vi "LogStatus.vi"(7 "Station":enum16{"A", "B"}(ring), 8 "error in (no error)":errorcluster, 9 "last message":string, 10 "message":string) -> (0 "error  out":errorcluster)   [LabVIEW 2017]
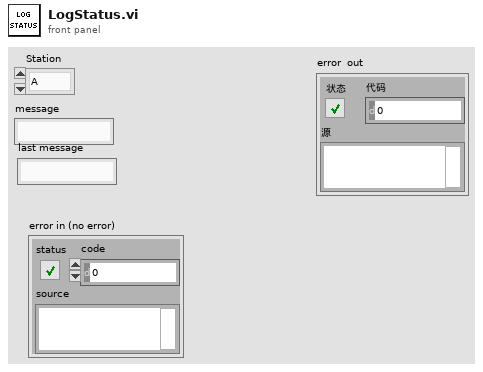
[diagram p1: front panel]
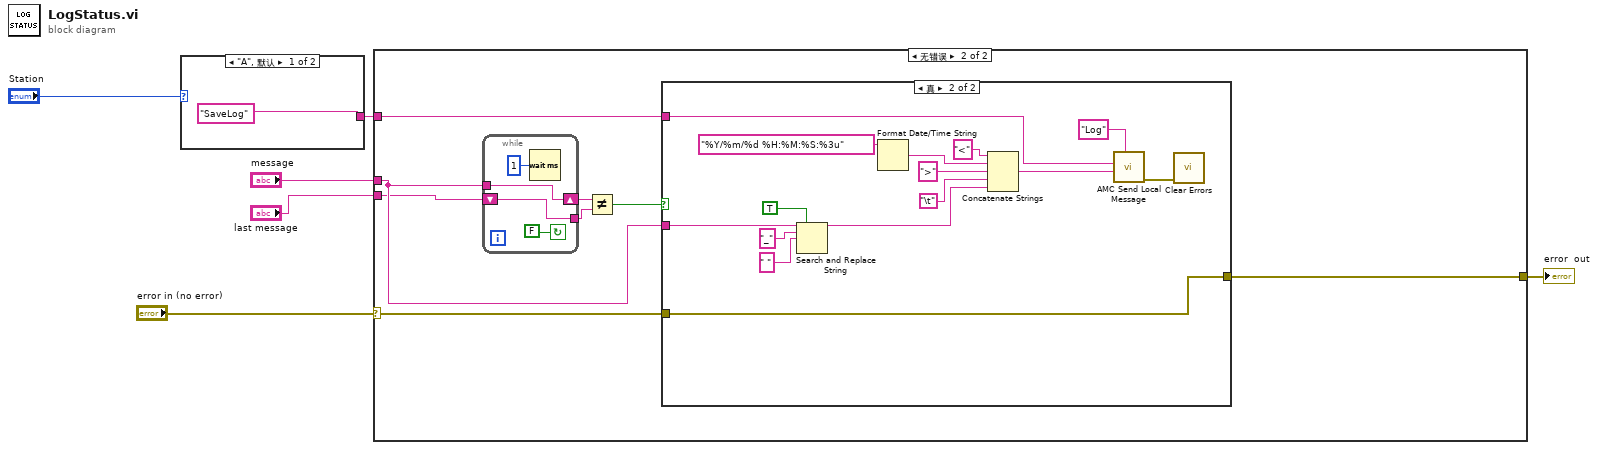
[diagram p0: block diagram]
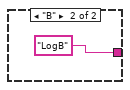
[diagram p2: hidden frame]
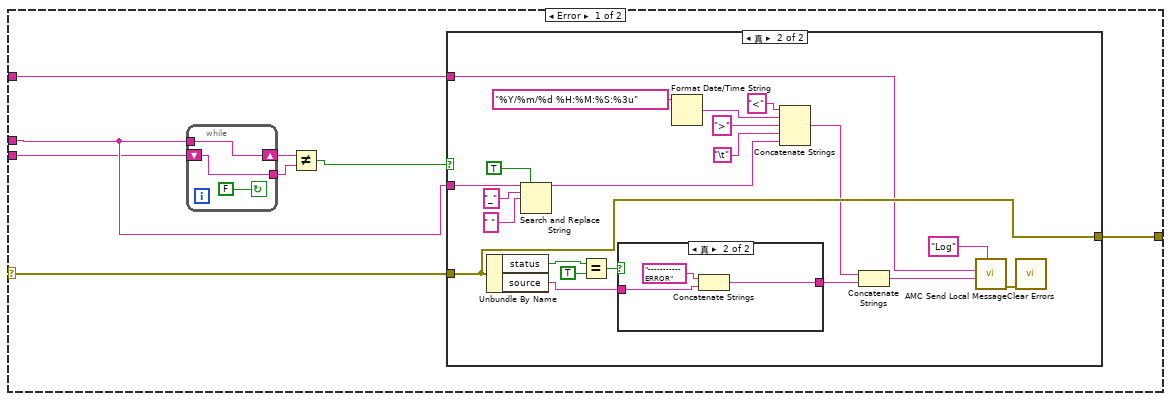
[diagram p3: hidden frame]
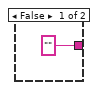
[diagram p5: hidden frame]
diagram:
  n1 = case shown="\"A\", 默认" "Station" {
    tunnel: ["SaveLog" ("Message Name") "LogB" ("Process (\"\" - local)")] -> w4
    frame "A", Default {
    }
    frame "B" {
    }
  }
  n2 = case shown="无错误" "error in (no error)" {
    selector: "error in (no error)" -> [w16 w53]
    tunnel: "message" -> [w11 w48]
    tunnel: [w15 w52] -> w6
    tunnel: w4 -> [w12 w51]
    tunnel: "last message" -> [w10 w47]
    frame Error {
      n3 = while {
        shift-right: [w19] -> w13
        shift-left: w10 -> [w18]
        tunnel: w11 -> [w19]
        tunnel: [w18] -> w14
        stop <- FALSE continue-if-true
      }
      n4 = Not Equal?(x=w13, y=w14) -> (x != y?=w9:bool)
      n5 = case shown="真" w9 {
        tunnel: w11 -> [_ w33]
        tunnel: w16 -> [w20 w32]
        tunnel: [w20 w32] -> w15
        tunnel: w12 -> [_ w22]
        frame False {
        }
        frame True {
          n6 = Unbundle By Name(w32) -> ("status"=w38:bool, "source"=w41:string)
          n7 = Search and Replace String(replace all?=TRUE ("替换全部？(F)"), input string=w33, search string="_" ("搜索字符串"), replace string=" " ("替换字符串(\"\")")) -> (result string=w25:string)  [unwired: 4 in, 3 out]
          n8 = Equal?(x=w38, y=TRUE) -> (x = y?=w40:bool)
          n9 = case shown="真" w40 {
            tunnel: ["" ("string") w44] -> w39
            tunnel: w41 -> [_ w43]
            frame False {
            }
            frame True {
              n10 = Concatenate Strings("-----------ERROR" ("string"), w43) -> (w44:string)
            }
          }
          n11 = Format Date/Time String(time format string (%c)="%Y/%m/%d %H:%M:%S:%3u" ("时间格式字符串(%c)")) -> (date/time string=w30:string)  [unwired: 2 in]
          n12 = Concatenate Strings("<" ("字符串"), w30, ">" ("字符串"), "\t", w25) -> (w24:string)
          n13 = Concatenate Strings(w24, w39) -> (w31:string)
          n14 = call "AMC Send Local Message.vi"("Process (\"\" - local)"="Log" ("Process (\"\" - local)"), "Message Value"=w31, "Message Name"=w22) -> ("error out"=w21:errorcluster)  [unwired: 7 in, 1 out]
          n15 = call <vilib>:"Clear Errors.vi"("error in (no error)"=w21) -> ()  [unwired: 5 in, 2 out]
        }
      }
    }
    frame No Error {
      n16 = while {
        shift-right: [w57] -> w49
        shift-left: w47 -> [w56]
        tunnel: w48 -> [w57]
        tunnel: [w56] -> w50
        stop <- FALSE continue-if-true
        n17 = Wait (ms)(milliseconds to wait=u32 1 ("等待时间（毫秒）")) -> ()  [unwired: 1 out]
      }
      n18 = Not Equal?(x=w49, y=w50) -> (x != y?=w46:bool)
      n19 = case shown="真" w46 {
        tunnel: w48 -> [_ w70]
        tunnel: w53 -> [w58 w69]
        tunnel: [w58 w69] -> w52
        tunnel: w51 -> [_ w60]
        frame False {
        }
        frame True {
          n20 = Search and Replace String(replace all?=TRUE ("替换全部？(F)"), input string=w70, search string="_" ("搜索字符串"), replace string=" " ("替换字符串(\"\")")) -> (result string=w63:string)  [unwired: 4 in, 3 out]
          n21 = Format Date/Time String(time format string (%c)="%Y/%m/%d %H:%M:%S:%3u" ("时间格式字符串(%c)")) -> (date/time string=w68:string)  [unwired: 2 in]
          n22 = Concatenate Strings("<" ("字符串"), w68, ">" ("字符串"), "\t", w63) -> (w62:string)
          n23 = call "AMC Send Local Message.vi"("Process (\"\" - local)"="Log" ("Message Name"), "Message Value"=w62, "Message Name"=w60) -> ("error out"=w59:errorcluster)  [unwired: 7 in, 1 out]
          n24 = call <vilib>:"Clear Errors.vi"("error in (no error)"=w59) -> ()  [unwired: 5 in, 2 out]
        }
      }
    }
  }
  "error  out" <- w6
